vi "PXI-Set Counter Config.vi"(0 "AI Sampling Rate (Hz)":dbl, 1 "Delay (ms)":dbl, 3 "pulse duration (ms)":dbl=0.25, 5 "Num AI Pts":i32, 11 "error in (no error)":errorcluster, 12 "Configure? (T)":bool=TRUE) -> (15 "error out":errorcluster)   [LabVIEW 2020]
uses:
  DAQ Engine VIs/PXI Globals.vi
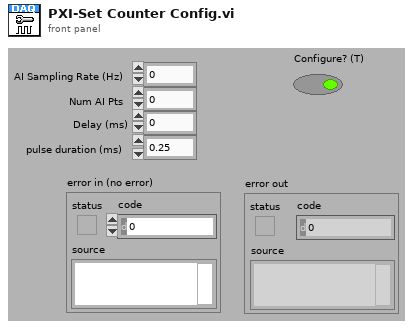
[diagram p1: front panel]
types:
  T1 = typedef "Counter Params.ctl" = cluster{"Counter":tag, "Hi ticks":u32, "Low ticks":u32, "Idle state":i32, "Delay ticks":u32}
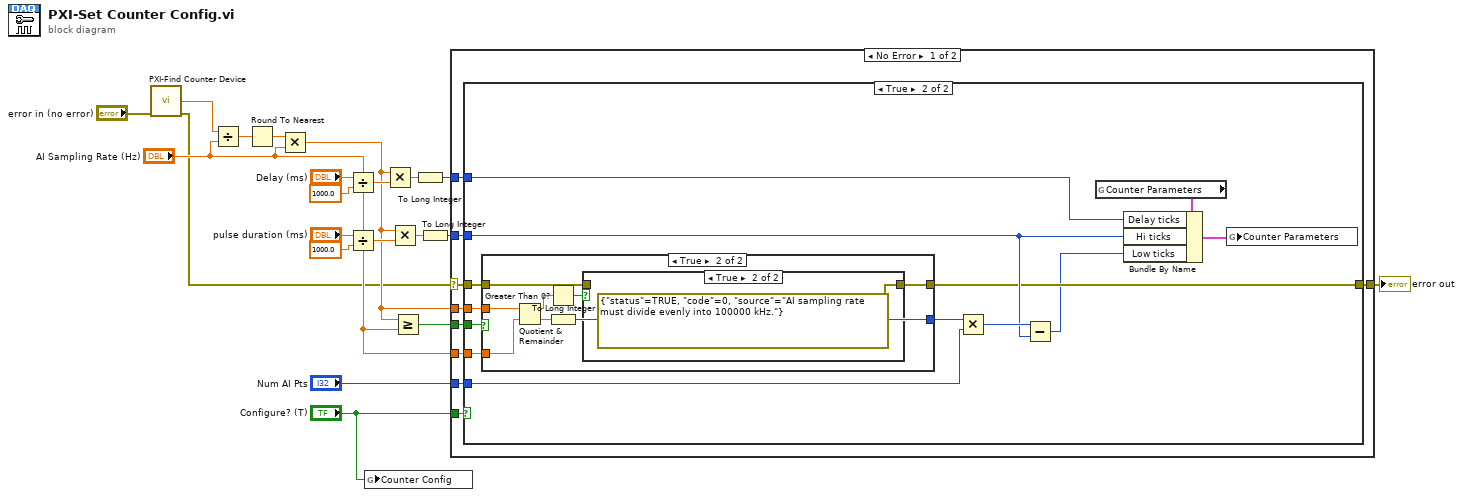
[diagram p0: block diagram]
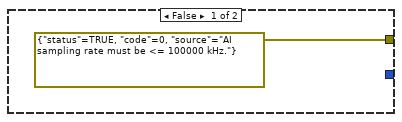
[diagram p3: hidden frame]
diagram:
  n1 = call "PXI-Find Counter Device.vi"("error in (no error)"="error in (no error)") -> ("Clock Rate"=w3:dbl, "error out"=w1:errorcluster)  [unwired: 10 in, 3 out]
  n2 = Divide(x=w3, y="AI Sampling Rate (Hz)") -> (x/y=w7:dbl)
  n3 = Round To Nearest(number=w7) -> (nearest integer value=w6:dbl)
  n4 = Multiply(x=w6, y="AI Sampling Rate (Hz)") -> (x*y=w4:dbl)
  n5 = Divide(x="Delay (ms)", y=1000.0) -> (x/y=w18:dbl)
  n6 = Divide(x="pulse duration (ms)", y=1000.0) -> (x/y=w13:dbl)
  n7 = global write "PXI Globals.vi" "Counter Config"("Configure? (T)") -> ()
  n8 = Multiply(x=w4, y=w18) -> (x*y=w20:dbl)
  n9 = Multiply(x=w4, y=w13) -> (x*y=w21:dbl)
  n10 = Greater Or Equal?(x=w4, y="AI Sampling Rate (Hz)") -> (x >= y?=w15:bool)
  n11 = To Long Integer(number=w20) -> (32bit integer=w11:i32)
  n12 = To Long Integer(number=w21) -> (32bit integer=w10:i32)
  n13 = case shown="No Error" w1 {
    selector: w1 -> [w22 w56]
    tunnel: w15 -> [w30 _]
    tunnel: "Num AI Pts" -> [w29 _]
    tunnel: w11 -> [w28 _]
    tunnel: w10 -> [w27 _]
    tunnel: [w26 w56] -> w9
    tunnel: "Configure? (T)" -> [w25 _]
    tunnel: "AI Sampling Rate (Hz)" -> [w24 _]
    tunnel: w4 -> [w23 _]
    frame No Error {
      n14 = case shown="True" w25 {
        tunnel: w30 -> [_ w44]
        tunnel: w23 -> [_ w43]
        tunnel: w24 -> [_ w42]
        tunnel: w29 -> [_ w40]
        tunnel: w22 -> [w31 w38]
        tunnel: w28 -> [_ w36]
        tunnel: w27 -> [_ w35]
        tunnel: [w31 w34] -> w26
        frame False {
        }
        frame True {
          n15 = case shown="True" w44 {
            tunnel: w43 -> [_ w53]
            tunnel: w42 -> [_ w52]
            tunnel: [_ w50] -> w39
            tunnel: w38 -> [_ w47]
            tunnel: [errorcluster {"status"=TRUE, "code"=0, "source"="AI sampling rate must be <= 100000 kHz."} ("error in (no error)") w46] -> w34
            frame False {
            }
            frame True {
              n16 = Quotient & Remainder(x=w53, y=w52) -> (x-y*floor(x/y)=w48:dbl, floor(x/y)=w51:dbl)
              n17 = Greater Than 0?(x=w48) -> (x > 0?=w49:bool)
              n18 = To Long Integer(number=w51) -> (32bit integer=w50:i32)
              n19 = case shown="True" w49 {
                tunnel: w47 -> [w54 _]
                tunnel: [w54 errorcluster {"status"=TRUE, "code"=0, "source"="AI sampling rate must divide evenly into 100000 kHz."} ("error in (no error)")] -> w46
                frame False {
                }
                frame True {
                }
              }
            }
          }
          n20 = Multiply(x=w39, y=w40) -> (x*y=w41:i32)
          n21 = Subtract(x=w41, y=w35) -> (x-y=w33:i32)
          n22 = global read "PXI Globals.vi" "Counter Parameters"() -> (w37:T1)
          n23 = Bundle By Name(cluster=w37, "Delay ticks"=w36, "Hi ticks"=w35, "Low ticks"=w33) -> (w32:T1)
          n24 = global write "PXI Globals.vi" "Counter Parameters"(w32) -> ()
        }
      }
    }
    frame Error {
    }
  }
  "error out" <- w9
